vi "Reciev_CANATII.vi"(3 "Display":bool, 4 "queue out":refnum<queue>, 5 "cnd_in":u32, 6 "Config":refnum<vi>) -> (0 "Data":u8[](array[numeric]), 1 "Sts":bool, 2 "cnt_out":u32)   [LabVIEW 2017]
uses:
  CAN TxRx/CAN/CANalystII/PCAN_Driver/ControlCAN.lvlib
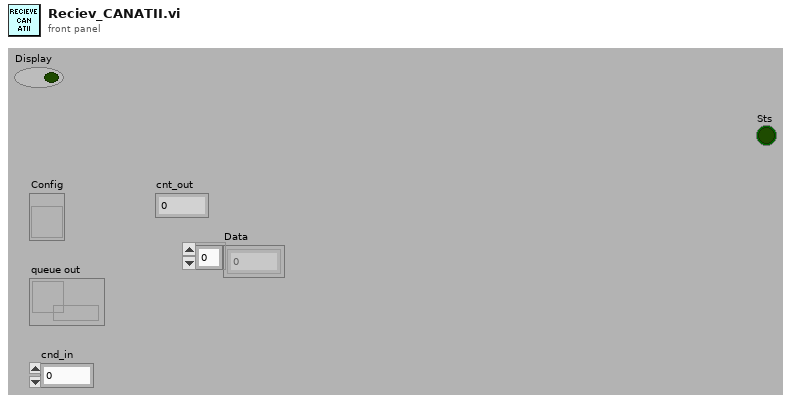
[diagram p1: front panel]
types:
  T1 = typedef "ControlCAN.lvlib/DevType.ctl" = u32
  T2 = typedef "ControlCAN.lvlib/CAN Channel.ctl" = u32
  T3 = typedef "ControlCAN.lvlib/VCI_INIT_CONFIG.ctl" = cluster{"AccCode":u32, "AccMask":u32, "InitFlag":T4, "Fliter":T5, "Timing0":u8, "Timing1":u8, "Mode":T6}
  T4 = typedef "ControlCAN.lvlib/InitFlag.ctl" = u32
  T5 = typedef "ControlCAN.lvlib/Fliter.ctl" = u8
  T6 = typedef "ControlCAN.lvlib/Mode.ctl" = u8
  T7 = cluster{"DevType":T1, "DevIndex":u32, "CanIndex":T2, "VCI_INIT_CONFIG":T3}
  T8 = typedef "ControlCAN.lvlib/VCI_CAN_OBJ.ctl" = cluster{"ID":u32, "TimeStamp":u32, "TimeFlag":u8, "SendType":u8, "RemoteFlag":u8, "ExternFlag":u8, "DataLen":u8, "Data":u8[], "Reserved":u8[]}
  T9 = cluster{"ID":u32, "MSGTYPE":u8, "LEN":u8, "aDATA":u8[]}
  T10 = cluster{"Type":enum16{"接收", "发送"}, "Channel":T2, "Time":timestamp, "VCI_CAN_OBJ":T8}[]
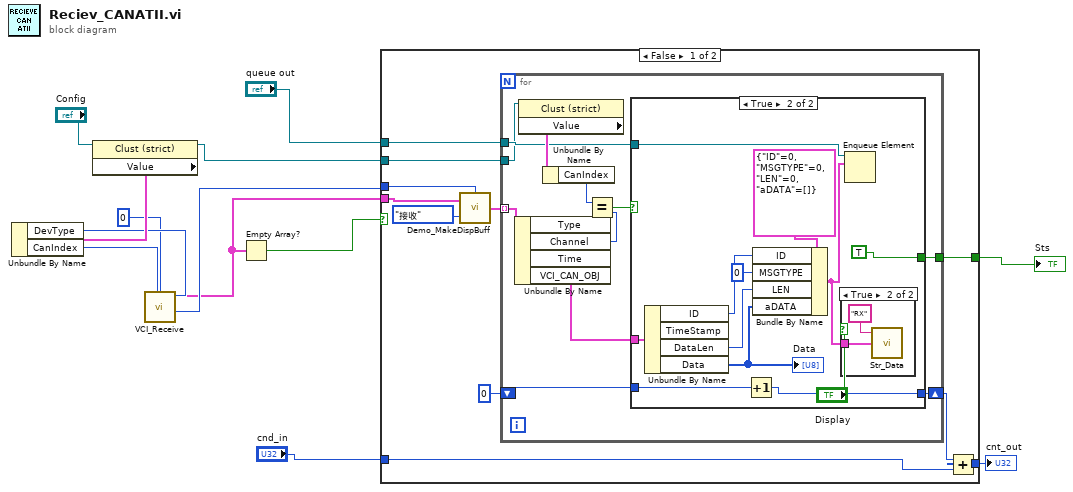
[diagram p0: block diagram]
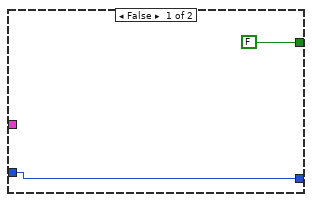
[diagram p2: hidden frame]
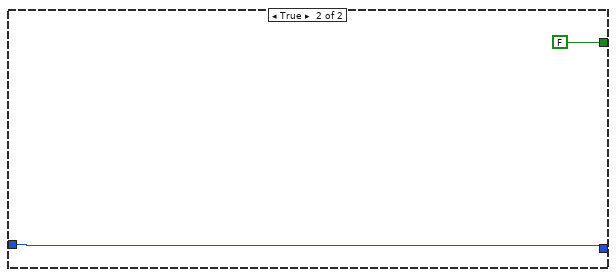
[diagram p4: hidden frame]
diagram:
  n1 = property class="Clust (strict)"(reference="Config") -> (reference out=w2:refnum<vi>, "Value"=w9:T7)  [unwired: 1 in, 1 out]
  n2 = Unbundle By Name(w9) -> ("DevType"=w7:T1, "CanIndex"=w8:T2)
  n3 = call "VCI_Receive.vi"("CANIndex"=w8, "DevIndex"=u32 0, "DevType"=w7) -> ("Recieve"=w6:T8[])  [unwired: 3 in, 5 out]
  n4 = Empty Array?(array=w6) -> (empty?=w5:bool)
  n5 = case shown="False" w5 {
    tunnel: w6 -> [w21 _]
    tunnel: w8 -> [w22 _]
    tunnel: "cnd_in" -> [w17 w52]
    tunnel: [w16 w52] -> w10
    tunnel: "queue out" -> [w15 _]
    tunnel: w2 -> [w14 _]
    tunnel: [w13 FALSE] -> w1
    frame False {
      n6 = call "Demo_MakeDispBuff.vi"("Channel"=w22, "Type"=enum16{"接收", "发送"}."接收", "OBJs"=w21) -> ("Buffer"=w20:T10)
      n7 = for {
        tunnel: w20 -> [w34] mode=indexing
        tunnel: w15 -> [w26]
        shift-right: [w27] -> w18
        shift-left: u32 0 -> [w28]
        tunnel: w14 -> [w25]
        tunnel: [w24] -> w13
        n8 = Unbundle By Name(w34) -> ("Channel"=w30:T2, "VCI_CAN_OBJ"=w33:T8)  [unwired: 2 out]
        n9 = property class="Clust (strict)"(reference=w25) -> ("Value"=w32:T7)  [unwired: 1 in, 2 out]
        n10 = Unbundle By Name(w32) -> ("CanIndex"=w31:T2)
        n11 = Equal?(x=w31, y=w30) -> (x = y?=w29:bool)
        n12 = case shown="True" w29 {
          tunnel: w26 -> [_ w41]
          tunnel: w33 -> [_ w47]
          tunnel: w28 -> [w36 w43]
          tunnel: [w36 w42] -> w27
          tunnel: [FALSE TRUE] -> w24
          frame False {
          }
          frame True {
            n13 = Unbundle By Name(w47) -> ("ID"=w46:u32, "DataLen"=w45:u8, "Data"=w44:u8[])  [unwired: 1 out]
            "Data" <- w44
            n14 = Increment(x=w43) -> (x+1=w42:u32)
            n15 = Bundle By Name(cluster=T9 {"ID"=0, "MSGTYPE"=0, "LEN"=0, "aDATA"=[]} ("Msg"), "ID"=w46, "MSGTYPE"=u8 0, "LEN"=w45, "aDATA"=w44) -> (w40:T9)
            n16 = case shown="True" "Display" {
              tunnel: w40 -> [_ w49]
              frame False {
              }
              frame True {
                n17 = call "Str_Data.vi"("Msg"=w49, "string"="RX") -> ()  [unwired: 1 in, 1 out]
              }
            }
            n18 = Enqueue Element(queue=w41, element=w40) -> ()  [unwired: 1 in, 4 out]
          }
        }
      }
      n19 = Add(x=w18, y=w17) -> (x+y=w16:u32)
    }
    frame True {
    }
  }
  "cnt_out" <- w10
  "Sts" <- w1
